vi "Turn Smother.vi"(2 "Ignore Deceleration":bool, 3 "Ignore Acceleration":bool, 4 "internal path stuff":T7 {"?"."Limits"."StoopidFast (fps)" min=0.0; "?"."Limits"."Jerk (fps^3)" min=0.0 step=1.0; "?"."Limits"."Accel (fps^2)" min=0.0; "?"."Limits"."Velocity (fps)" min=0.0; "?"."Overrides"."Angle Override" step=5.0; "?"."Overrides"."Velocity Override" step=5.0; "?"."Overrides"."Angular Override" step=5.0; "?"."Angular Limits"."Jerk (deg/s^3)" min=0.0 step=1.0; "?"."Angular Limits"."Accel (deg/s^2)" min=0.0; "?"."Angular Limits"."Velocity (deg/s)" min=0.0}) -> (1 "Overrides":T3 {"Angle Override" step=5.0; "Velocity Override" step=5.0; "Angular Override" step=5.0})   [LabVIEW 2025]
uses:
  Types/Overrides.ctl
  Types/Segment Type.ctl
  Types/Limits.ctl
  Types/Angluar Limits.ctl
  Types/Single Cmd Info.ctl
  <vilib>/picture/picture.llb/imagedata.ctl
panel:
  out "Array":bool[](array[boolean])
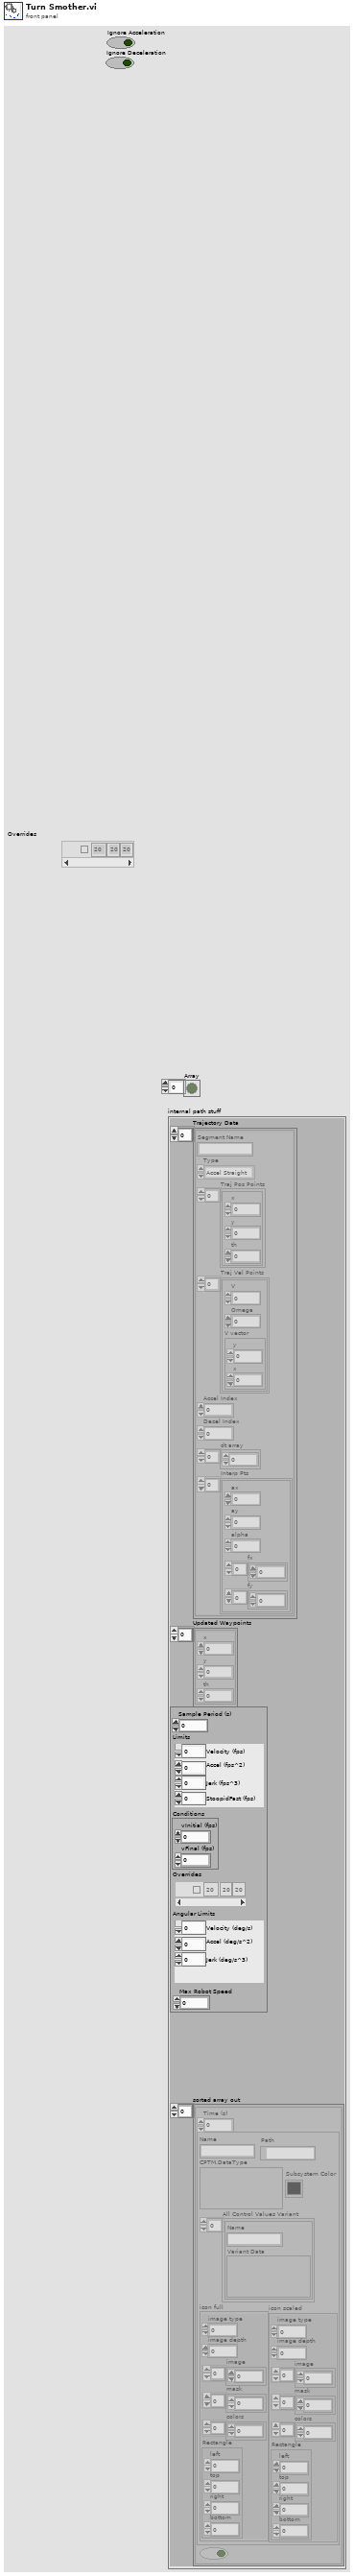
[diagram p1: front panel]
types:
  T1 = typedef "Segment Type.ctl" = enum16{"Accel Straight", "Const Straight", "Blend", "Circle", "Bezier", "Choreo"}
  T2 = typedef "Limits.ctl" = cluster{"Velocity (fps)":dbl, "Accel (fps^2)":dbl, "Jerk (fps^3)":dbl, "StoopidFast (fps)":dbl}
  T3 = typedef "Overrides.ctl" = cluster{"Count":string, "Angular Override":dbl, "Enabled?":bool, "Velocity Override":dbl, "Angle Override":dbl}[]
  T4 = typedef "Angluar Limits.ctl" = cluster{"Velocity (deg/s)":dbl, "Accel (deg/s^2)":dbl, "Jerk (deg/s^3)":dbl}
  T5 = typedef "Single Cmd Info.ctl" = cluster{"Name":string, "CPTM.DataType":variant, "All Control Values Variant":cluster{"Name":string, "Variant Data":variant}[], "icon full":T6, "icon scaled":T6, "Path":path, "Subsystem Color":u32}
  T6 = typedef "imagedata.ctl" = cluster{"image type":i32, "image depth":i32, "image":u8[], "mask":u8[], "colors":u32[], "Rectangle":cluster{"left":i16, "top":i16, "right":i16, "bottom":i16}}
  T7 = cluster{"Trajectory Data":cluster{"Segment Name":string, "Type":T1, "Traj Pos Points":cluster{"x":dbl, "y":dbl, "th":dbl}[], "Traj Vel Points":cluster{"V":dbl, "Omega":dbl, "V vector":cluster{"y":dbl, "x":dbl}}[], "Accel Index":i32, "Decel Index":i32, "dt array":dbl[], "Interp Pts":cluster{"ax":dbl, "ay":dbl, "alpha":dbl, "fx":dbl[], "fy":dbl[]}[]}[], "Updated Waypoints":cluster{"x":dbl, "y":dbl, "th":dbl}[], cluster{"Sample Period (s)":dbl, "Limits":T2, "Conditions":cluster{"vInitial (fps)":dbl, "vFinal (fps)":dbl}, "Overrides":T3, "Angular Limits":T4, "Max Robot Speed":dbl}, "sorted array out":cluster{"Time (s)":dbl, T5, bool}[]}
  T8 = cluster{"Segment Name":string, "Type":T1, "Traj Pos Points":cluster{"x":dbl, "y":dbl, "th":dbl}[], "Traj Vel Points":cluster{"V":dbl, "Omega":dbl, "V vector":cluster{"y":dbl, "x":dbl}}[], "Accel Index":i32, "Decel Index":i32, "dt array":dbl[], "Interp Pts":cluster{"ax":dbl, "ay":dbl, "alpha":dbl, "fx":dbl[], "fy":dbl[]}[]}[]
  T9 = cluster{"Sample Period (s)":dbl, "Limits":T2, "Conditions":cluster{"vInitial (fps)":dbl, "vFinal (fps)":dbl}, "Overrides":T3, "Angular Limits":T4, "Max Robot Speed":dbl}
  T10 = cluster{"vInitial (fps)":dbl, "vFinal (fps)":dbl}
  T11 = cluster{string, dbl, bool, "Velocity (fps)":dbl, dbl}
  T12 = cluster{string, dbl, bool, "Velocity (fps)":dbl, dbl}[]
  T13 = cluster{"Segment Name":string, "Type":T1, "Traj Pos Points":cluster{"x":dbl, "y":dbl, "th":dbl}[], "Traj Vel Points":cluster{"V":dbl, "Omega":dbl, "V vector":cluster{"y":dbl, "x":dbl}}[], "Accel Index":i32, "Decel Index":i32, "dt array":dbl[], "Interp Pts":cluster{"ax":dbl, "ay":dbl, "alpha":dbl, "fx":dbl[], "fy":dbl[]}[]}
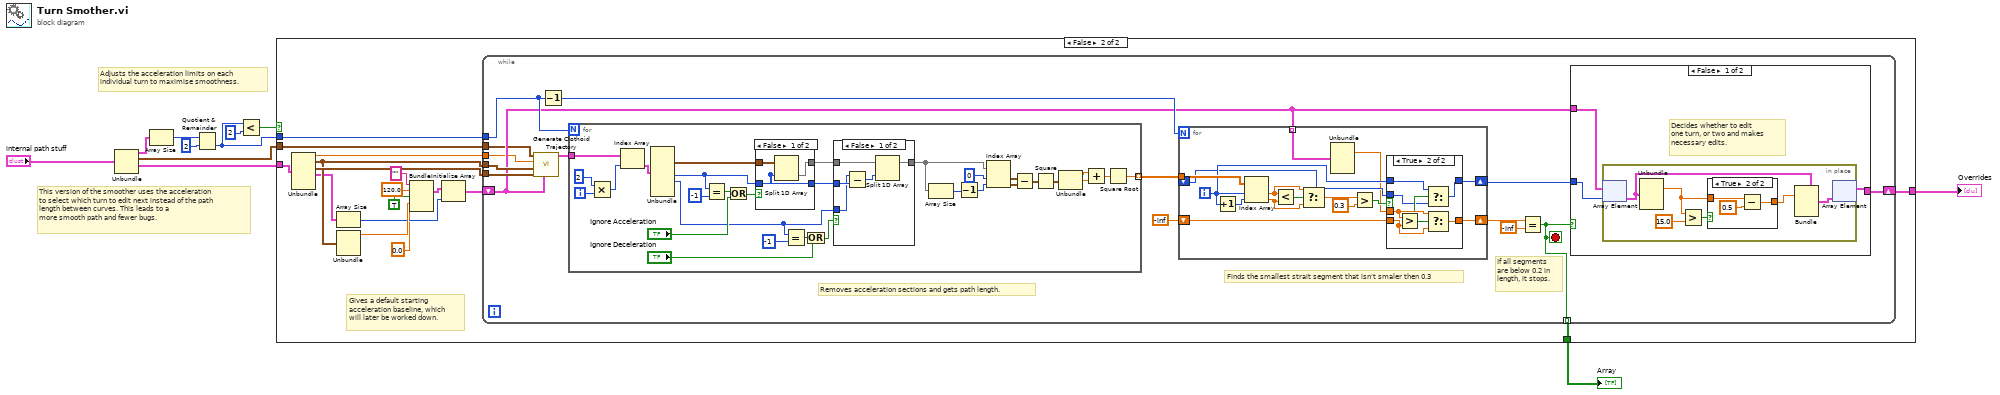
[diagram p0: block diagram]
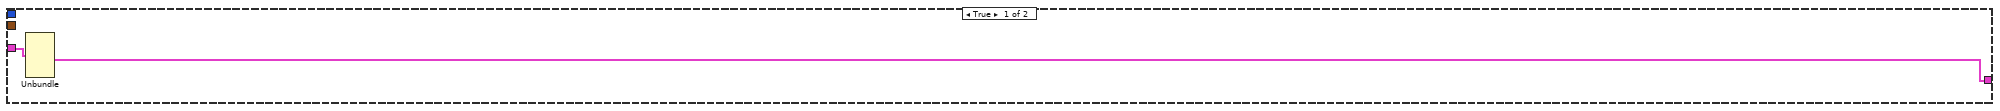
[diagram p2: hidden frame]
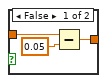
[diagram p3: hidden frame]
diagram:
  # "This version of the smoother uses the acceleration\nto select which turn to edit next instead of the path \nlength between curves. This leads to a \nmore smooth path and fewer bugs."
  # "Adjusts the acceleration limits on each \nindividual turn to maximise smoothness."
  n1 = Unbundle("internal path stuff") -> ("Trajectory Data"=w5:T8, "Updated Waypoints"=w4:cluster{"x":dbl, "y":dbl, "th":dbl}[], w6:T9)  [unwired: 1 out]
  n2 = Array Size(array=w5) -> (size(s)=w11:i32)
  n3 = Quotient & Remainder(x=w11, y=2) -> (floor(x/y)=w8:i32)  [unwired: 1 out]
  n4 = Less?(x=w8, y=2) -> (x < y?=w7:bool)
  n5 = case shown="False" w7 {
    tunnel: w8 -> [_ w30]
    tunnel: [w13 w29] -> w3
    tunnel: w6 -> [w12 w28]
    tunnel: w4 -> [_ w26]
    tunnel: [_ w14] -> w2
    frame True {
      n6 = Unbundle(w12) -> ("Overrides"=w13:T3)  [unwired: 5 out]
    }
    frame False {
      # "Gives a default starting \nacceleration baseline, which\nwill later be worked down."
      n7 = Unbundle(w28) -> ("Sample Period (s)"=w27:dbl, "Limits"=w24:T2, "Conditions"=w25:T10, "Overrides"=w23:T3)  [unwired: 2 out]
      n8 = Array Size(array=w23) -> (size(s)=w18:i32)
      n9 = Unbundle(w24) -> ("Velocity (fps)"=w19:dbl)  [unwired: 3 out]
      n10 = Bundle("", 120.0, TRUE, "Velocity (fps)"=w19, 0.0) -> (w17:T11)  [unwired: 1 in]
      n11 = Initialize Array(w17, w18) -> (w16:T12)
      n12 = while {
        shift-right: [w44] -> w29
        shift-left: w16 -> [w34]
        tunnel: w30 -> [w41]
        tunnel: w27 -> [w33]
        tunnel: w26 -> [w32]
        tunnel: w24 -> [w39]
        tunnel: w25 -> [w38]
        tunnel: [w31] -> w14 mode=indexing
        stop <- w31 stop-if-true
        # "If all segments\nare below 0.2 in\nlength, it stops."
        # "Removes acceleration sections and gets path length."
        # "Finds the smallest strait segment that isn't smaler then 0.3"
        n13 = call "Generate Clothoid Trajectory.vi"("Overrides"=w34, "Conditions"=w38, "Limits"=w39, "Sample Period (s)"=w33, "WayPoints"=w32) -> ("Traj Data"=w40:T8)  [unwired: 3 in, 3 out]
        n14 = Decrement(x=w41) -> (x-1=w42:i32)
        n15 = for {
          N: w41 -> [_]
          tunnel: w40 -> [w89]
          tunnel: [w79] -> w43 mode=indexing
          i -> [w91]
          n16 = Multiply(x=2, y=w91) -> (x*y=w88:i32)
          n17 = Index Array(array=w89, index=w88) -> (element=w87:T13)
          n18 = Unbundle(w87) -> ("Traj Pos Points"=w80:cluster{"x":dbl, "y":dbl, "th":dbl}[], "Accel Index"=w76:i32, "Decel Index"=w69:i32)  [unwired: 5 out]
          n19 = Equal?(x=w76, y=-1) -> (x = y?=w77:bool)
          n20 = Or(x=w77, y="Ignore Acceleration") -> (x .or. y?=w75:bool)
          n21 = case shown="False" w75 {
            tunnel: w80 -> [w100 w101]
            tunnel: [w99 w101] -> w86
            tunnel: [w98 _] -> w85
            tunnel: w76 -> [w98 _]
            frame False {
              n22 = Split 1D Array(array=w100, index=w98) -> (second subarray=w99:cluster{"x":dbl, "y":dbl, "th":dbl}[])  [unwired: 1 out]
            }
            frame True {
            }
          }
          n23 = Equal?(x=w69, y=-1) -> (x = y?=w72:bool)
          n24 = Or(x=w72, y="Ignore Deceleration") -> (x .or. y?=w70:bool)
          n25 = case shown="False" w70 {
            tunnel: w86 -> [w96 w97]
            tunnel: [w95 w97] -> w83
            tunnel: w85 -> [w94 _]
            tunnel: w69 -> [w92 _]
            frame False {
              n26 = Subtract(x=w92, y=w94) -> (x-y=w93:i32)
              n27 = Split 1D Array(array=w96, index=w93) -> (first subarray=w95:cluster{"x":dbl, "y":dbl, "th":dbl}[])  [unwired: 1 out]
            }
            frame True {
            }
          }
          n28 = Array Size(array=w83) -> (size(s)=w82:i32)
          n29 = Decrement(x=w82) -> (x-1=w81:i32)
          n30 = Index Array(array=w83, index #1=0 ("index"), index #2=w81) -> (element #1=w68:cluster{"x":dbl, "y":dbl, "th":dbl}, element #2=w67:cluster{"x":dbl, "y":dbl, "th":dbl})
          n31 = Subtract(x=w68, y=w67) -> (x-y=w66:cluster{"x":dbl, "y":dbl, "th":dbl})
          n32 = Square(x=w66) -> (x^2=w65:cluster{"x":dbl, "y":dbl, "th":dbl})
          n33 = Unbundle(w65) -> ("x"=w63:dbl, "y"=w64:dbl)  [unwired: 1 out]
          n34 = Add(x=w63, y=w64) -> (x+y=w62:dbl)
          n35 = Square Root(x=w62) -> (sqrt(x)=w79:dbl)
        }
        n36 = for {
          N: w42 -> [_]
          tunnel: w43 -> [w116]
          shift-right: [w111] -> w45
          shift-left: -inf -> [w110]
          tunnel: w34 -> [w103] mode=indexing
          shift-right: [w105] -> w35
          shift-left: _ -> [w104]
          i -> [w106]
          n37 = Increment(x=w106) -> (x+1=w115:i32)
          n38 = Index Array(array=w116, index #1=w106, index #2=w115) -> (element #1=w112:dbl, element #2=w113:dbl)
          n39 = Less?(x=w112, y=w113) -> (x < y?=w114:bool)
          n40 = Select(t=w112, s=w114, f=w113) -> (s? t:f=w108:dbl)
          n41 = Unbundle(w103) -> (w102:dbl)  [unwired: 4 out]
          n42 = Greater?(x=w108, y=0.3) -> (0:w109:bool)
          n43 = case shown="True" w109 {
            tunnel: [w118 w125] -> w111
            tunnel: w110 -> [w118 w124]
            tunnel: w102 -> [_ w123]
            tunnel: w106 -> [_ w121]
            tunnel: [w117 w119] -> w105
            tunnel: w104 -> [w117 w120]
            frame False {
            }
            frame True {
              n44 = Greater?(x=w123, y=w124) -> (0:w122:bool)
              n45 = Select(t=w121, s=w122, f=w120) -> (s? t:f=w119:i32)
              n46 = Select(t=w123, s=w122, f=w124) -> (s? t:f=w125:dbl)
            }
          }
        }
        n47 = Equal?(x=w45, y=-inf) -> (x = y?=w31:bool)
        n48 = case shown="False" w31 {
          tunnel: w34 -> [w46 w61]
          tunnel: [w47 w61] -> w44
          tunnel: w35 -> [w48 _]
          frame False {
            # "Decides whether to edit\none turn, or two and makes\nnecessary edits."
            n49 = in-place {
              n50 = in-place-array #1(w46, w48) -> (w51:T11)
              n51 = Unbundle(w51) -> (w52:dbl)  [unwired: 4 out]
              n52 = Greater?(x=w52, y=15.0) -> (0:w53:bool)
              n53 = case shown="True" w53 {
                tunnel: [w56 w59] -> w50
                tunnel: w52 -> [w57 w58]
                frame False {
                  n54 = Subtract(x=w57, y=0.05) -> (x-y=w56:dbl)
                }
                frame True {
                  n55 = Subtract(x=w58, y=0.5) -> (x-y=w59:dbl)
                }
              }
              n56 = Bundle(cluster=w51, w50) -> (w49:T11)  [unwired: 4 in]
              n57 = in-place-array #1(w49) -> (w47:T12)  [unwired: 1 out]
            }
          }
          frame True {
          }
        }
      }
    }
  }
  "Overrides" <- w3
  "Array" <- w2
